vi "Read Data.vi"(8 "error in (no error)":errorcluster caption="错误输入（无错误）", 11 "GPS 输入":refnum<class "GPS.lvclass">) -> (0 "error out":errorcluster caption="错误输出", 3 "GPS 输出":refnum<class "GPS.lvclass">)   [LabVIEW 2016, in "GPS.lvlib" / "GPS.lvclass"]
uses:
  GPS.lvclass
  GPS.lvclass/GPS.ctl
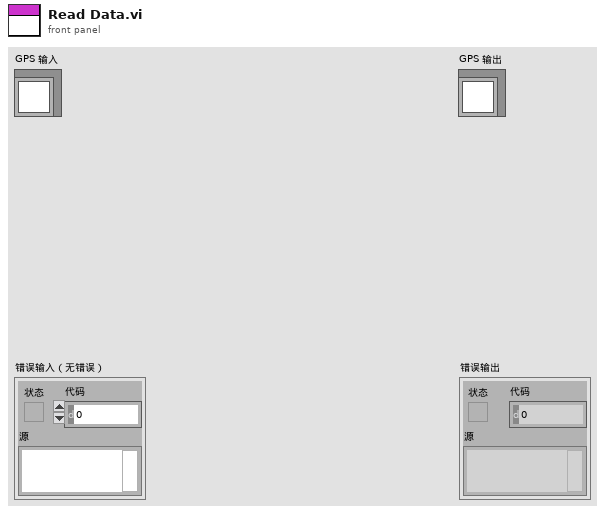
[diagram p1: front panel]
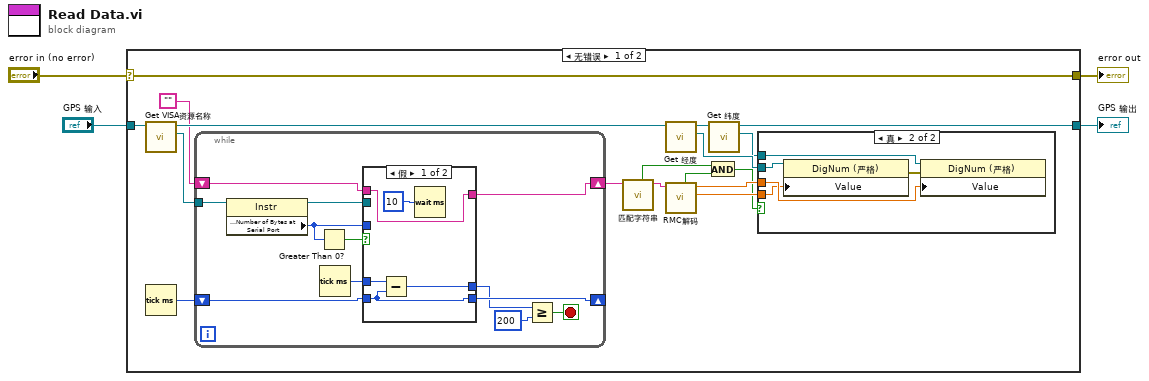
[diagram p0: block diagram]
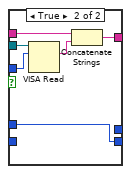
[diagram p3: hidden frame]
diagram:
  n1 = case shown="无错误" "error in (no error)" {
    selector: "error in (no error)" -> [w21 w51]
    tunnel: [w21 w51] -> w3
    tunnel: "GPS 输入" -> [w20 w50]
    tunnel: [w9 w50] -> w1
    frame No Error {
      n2 = call "Get VISA资源名称.vi"("GPS in"=w20) -> ("VISA资源名称"=w19:refnum<visa-resource-name>, "GPS out"=w15:refnum<class "GPS.lvclass">)  [unwired: 9 in]
      n3 = Tick Count (ms)() -> (millisecond timer value=w18:u32)
      n4 = while {
        tunnel: w19 -> [w38]
        shift-right: [w34] -> w16
        shift-left: "" -> [w33]
        shift-right: [w30] -> _
        shift-left: w18 -> [w32]
        stop <- w27 stop-if-true
        n5 = property class="Instr"(reference=w38) -> (reference out=w37:refnum<visa-resource-name>, "Serial Settings:Number of Bytes at Serial Port"=w36:u32)  [unwired: 1 in, 1 out]
        n6 = Greater Than 0?(x=w36) -> (x > 0?=w35:bool)
        n7 = Tick Count (ms)() -> (millisecond timer value=w31:u32)
        n8 = case shown="假" w35 {
          tunnel: w37 -> [_ w49]
          tunnel: w36 -> [_ w48]
          tunnel: [w42 w45] -> w34
          tunnel: w33 -> [w42 w47]
          tunnel: w32 -> [w40 _]
          tunnel: w31 -> [w41 w44]
          tunnel: [w40 w44] -> w30
          tunnel: [w39 _] -> w29
          frame False {
            n9 = Subtract(x=w41, y=w40) -> (x-y=w39:u32)
            n10 = Wait (ms)(milliseconds to wait=u32 10 ("等待时间（毫秒）")) -> ()  [unwired: 1 out]
          }
          frame True {
            n11 = VISA Read(VISA resource name=w49, byte count=w48) -> (read buffer=w46:string)  [unwired: 1 in, 3 out]
            n12 = Concatenate Strings(w47, w46) -> (w45:string)
          }
        }
        n13 = Greater Or Equal?(x=w29, y=u32 200) -> (x >= y?=w27:bool)
      }
      n14 = call "匹配字符串.vi"("字符串"=w16) -> ("所有匹配"=w17:string, "是否匹配？"=w7:bool)  [unwired: 9 in]
      n15 = call "Get 经度.vi"("GPS in"=w15) -> ("经度"=w13:refnum<vi>, "GPS out"=w14:refnum<class "GPS.lvclass">)  [unwired: 9 in]
      n16 = call "RMC解码.vi"("所有匹配"=w17) -> ("经度"=w10:dbl, "纬度"=w12:dbl, "定位OK?"=w6:bool)  [unwired: 8 in]
      n17 = And(x=w7, y=w6) -> (x .and. y?=w8:bool)
      n18 = call "Get 纬度.vi"("GPS in"=w14) -> ("纬度"=w11:refnum<vi>, "GPS out"=w9:refnum<class "GPS.lvclass">)  [unwired: 9 in]
      n19 = case shown="真" w8 {
        tunnel: w13 -> [_ w26]
        tunnel: w12 -> [_ w23]
        tunnel: w11 -> [_ w25]
        tunnel: w10 -> [_ w22]
        frame False {
        }
        frame True {
          n20 = property class="DigNum (严格)"(reference=w26, "Value"=w22) -> (error out=w24:errorcluster)  [unwired: 1 in, 1 out]
          n21 = property class="DigNum (严格)"(reference=w25, error in=w24, "Value"=w23) -> ()  [unwired: 2 out]
        }
      }
    }
    frame Error {
    }
  }
  "error out" <- w3
  "GPS 输出" <- w1
